vi "UpdateSequenceValuesTC.vi"(8 "error in (no error)":errorcluster, 9 "SignificantDigits (8)":u32=8, 10 "Format (SI notation)":T1(ring)=enum."SI notation", 11 "VMUI in":refnum<class "VMUI.lvclass">) -> (0 "error out":errorcluster, 3 "VMUI out":refnum<class "VMUI.lvclass">)   [LabVIEW 2013, in "VMUI.lvclass"]
uses:
  VMUI.lvclass
  <vilib>/Utility/miscctls.llb/LVRowAndColumnUnsignedTypeDef.ctl
  <vilib>/Utility/miscctls.llb/LVRowAndColumnTypeDef.ctl
  API/VariableManagerAPI.lvlib
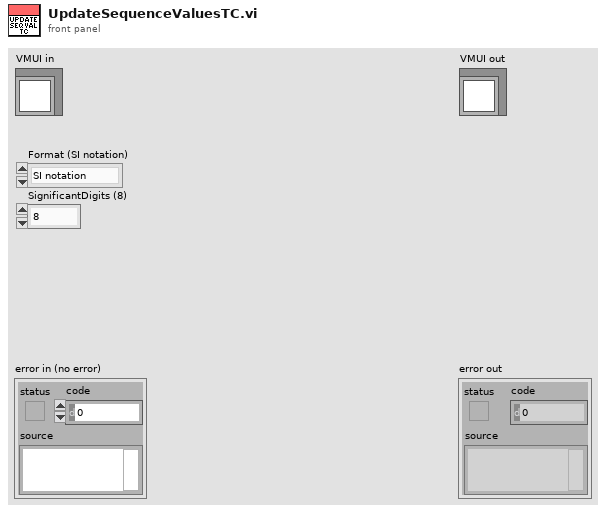
[diagram p1: front panel]
types:
  T1 = enum16{"Floating point", "Scientific SI", "Automatic SI", "SI notation"}
  T2 = typedef "LVRowAndColumnTypeDef.ctl" = cluster{"Row":i32, "Column":i32}
  T3 = typedef "LVRowAndColumnUnsignedTypeDef.ctl" = cluster{"Row":u32, "Column":u32}
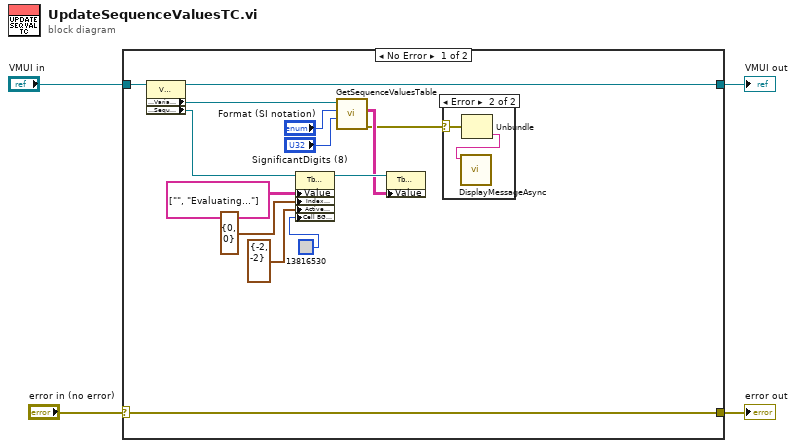
[diagram p0: block diagram]
diagram:
  n1 = case shown="No Error" "error in (no error)" {
    selector: "error in (no error)" -> [w17 w22]
    tunnel: [w17 w22] -> w3
    tunnel: [w12 w21] -> w1
    tunnel: "VMUI in" -> [w18 w21]
    frame No Error {
      n2 = property class="VMUI.lvclass"(reference=w18) -> (reference out=w12:refnum<class "VMUI.lvclass">, "Accessors:VariableManagerRef"=w10:refnum<vi>, "Accessors:SequenceValuesTCRef"=w11:refnum<vi>)  [unwired: 1 in, 1 out]
      n3 = property class="Tbl (strict)"(reference=w11, "Value"=string[][] [["", "Evaluating..."]], "Index Values"=T3 {"Row"=0, "Column"=0}, "Active Cell"=T2 {"Row"=-2, "Column"=-2} ("Active Cell:Active Cell"), "Cell BG Color"=u32 13816530) -> (reference out=w7:refnum<vi>)  [unwired: 1 in, 1 out]
      n4 = call "GetSequenceValuesTable.vi"("SignificantDigits (8)"="SignificantDigits (8)", "Format (SI notation)"="Format (SI notation)", "VariableManagerRef in"=w10) -> ("error out"=w5:errorcluster, "SequenceValuesTable"=w6:string[][])  [unwired: 6 in, 1 out]
      n5 = property class="Tbl (strict)"(reference=w7, "Value"=w6) -> ()  [unwired: 1 in, 2 out]
      n6 = case shown="Error" w5 {
        selector: w5 -> [_ w20]
        frame No Error {
        }
        frame Error {
          n7 = Unbundle(w20) -> ("source"=w19:string)  [unwired: 2 out]
          n8 = call "DisplayMessageAsync.vi"("Message"=w19) -> ()  [unwired: 11 in]
        }
      }
    }
    frame Error {
    }
  }
  "error out" <- w3
  "VMUI out" <- w1
